vi "(SUBVI) - Material.vi"(10 "Port (Port 1)":T2 items=["Port 1", "Port 2", "Port 3", "Port 4"], 11 "NXT/EV3":T1) -> (2 "Scaled dif":dbl, 3 "NXT/EV3 2":T1)   [LabVIEW 2016]
uses:
  <vilib>/NXT/Block Support/NXT_InputPort.ctl
  <vilib>/NXT/Subs/LVHSConnector.ctl
  <vilib>/NXT/LegoClasses/BrickReference/BrickReference.lvclass
  <vilib>/NXT/Dual Mode Library/Display/drawText.vi
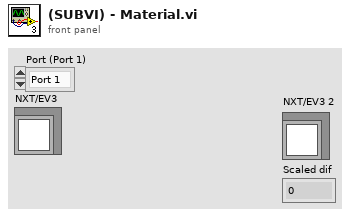
[diagram p1: front panel]
types:
  T1 = typedef "LVHSConnector.ctl" = refnum<class "BrickReference.lvclass">
  T2 = typedef "NXT_InputPort.ctl" = u32
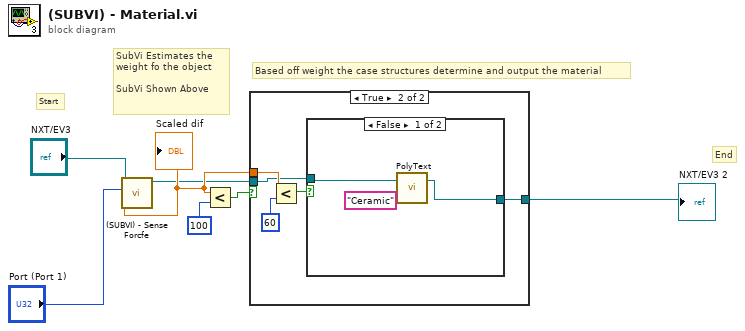
[diagram p0: block diagram]
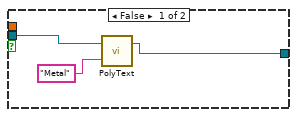
[diagram p2: hidden frame]
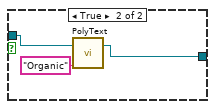
[diagram p3: hidden frame]
diagram:
  # "End"
  # "Based off weight the case structures determine and output the material"
  # "SubVi Estimates the weight fo the object\n\nSubVi Shown Above"
  # "Start"
  n1 = call "(SUBVI) - Sense Forcfe.vi"("Port (Port 1)"="Port (Port 1)", "NXT/EV3"="NXT/EV3") -> ("NXT/EV3 2"=w1:T1, "Scaled dif"=w3:dbl)  [unwired: 7 in, 1 out]
  "Scaled dif" <- w3
  n2 = Less?(x=w3, y=100) -> (x < y?=w4:bool)
  n3 = case shown="True" w4 {
    tunnel: w1 -> [w10 w12]
    tunnel: [w8 w11] -> w2
    tunnel: w3 -> [_ w15]
    frame False {
      n4 = call-poly <vilib>:"PolyText.vi"("Text"="Metal", "NXT/EV3"=w10) -> ("NXT/EV3"=w8:T1)  [unwired: 2 in]
    }
    frame True {
      n5 = Less?(x=w15, y=60) -> (x < y?=w14:bool)
      n6 = case shown="False" w14 {
        tunnel: w12 -> [w17 w21]
        tunnel: [w16 w20] -> w11
        frame False {
          n7 = call-poly <vilib>:"PolyText.vi"("Text"="Ceramic", "NXT/EV3"=w17) -> ("NXT/EV3"=w16:T1)  [unwired: 2 in]
        }
        frame True {
          n8 = call-poly <vilib>:"PolyText.vi"("Text"="Organic", "NXT/EV3"=w21) -> ("NXT/EV3"=w20:T1)  [unwired: 2 in]
        }
      }
    }
  }
  "NXT/EV3 2" <- w2
